vi "Build Frame Script Core.vi"(8 "error in (no error)":errorcluster, 10 "Config Array":string[](array[string]), 11 "Protocol Interface in":refnum<class "Protocol Interface.lvclass">) -> (0 "error out":errorcluster, 2 "Pattern Script":string, 3 "Protocol Interface out":refnum<class "Protocol Interface.lvclass">)   [LabVIEW 2018, in "Protocol Interface.lvlib" / "Protocol Interface.lvclass"]
uses:
  Protocol Interface.lvclass
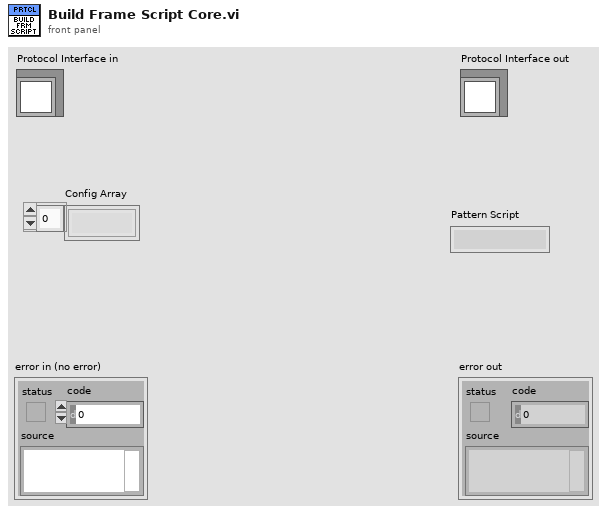
[diagram p1: front panel]
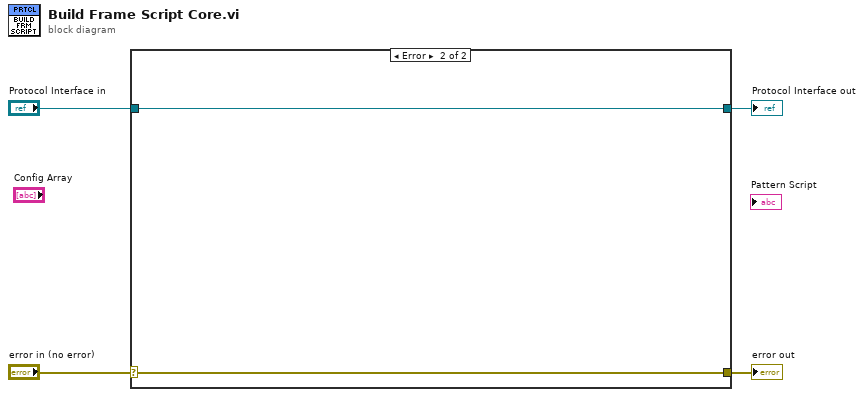
[diagram p0: block diagram]
diagram:
  n1 = case shown="Error" "error in (no error)" {
    selector: "error in (no error)" -> [w5 w8]
    tunnel: [w5 w8] -> w3
    tunnel: [w6 w7] -> w1
    tunnel: "Protocol Interface in" -> [w6 w7]
    frame No Error {
    }
    frame Error {
    }
  }
  "error out" <- w3
  "Protocol Interface out" <- w1
